vi "Result Calculation.vi"(10 "Frequency List":T1(array[cluster]), 11 "Fundamental-Response":T2(graph) caption="Fundamental-Response Mic1") -> (2 "Sensitivity Frequency (Hz)":dbl, 3 "Sensitivity (dBSPL)":dbl, 5 "Processed Freq Response":T2(graph) caption="Fundamental-Response Mic1", 7 "ProcessedFrequencyResponse":dbl[](array[numeric]))   [LabVIEW 2018]
panel:
  # "Result Calculation"
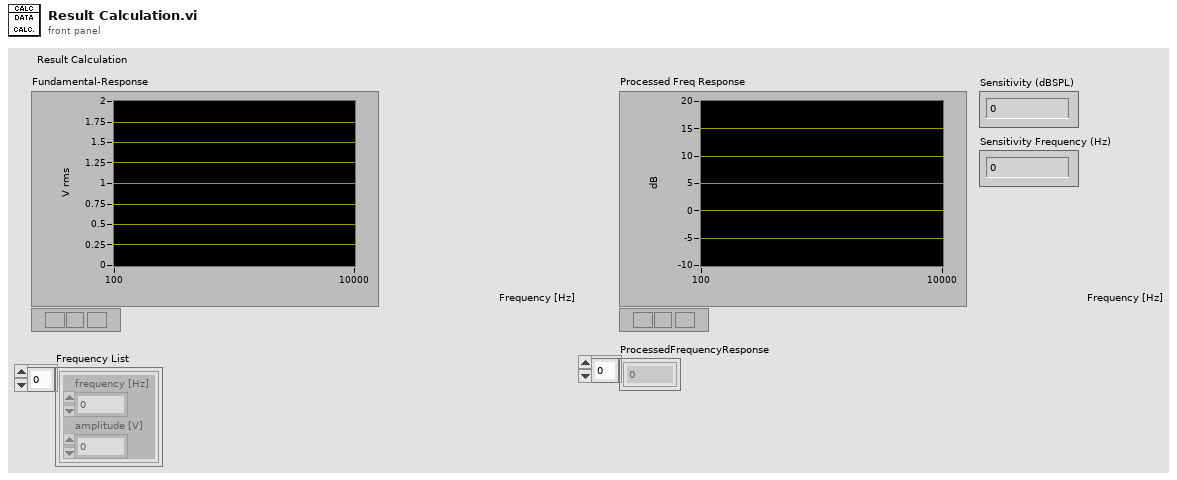
[diagram p1: front panel]
types:
  T1 = cluster{"frequency [Hz]":dbl, "amplitude [V]":dbl}[]
  T2 = cluster{"frequency [Hz]":dbl[], "amplitude":dbl[]}
  T3 = cluster{"frequency [Hz]":dbl[], "ProcessedFrequencyResponse":dbl[]}
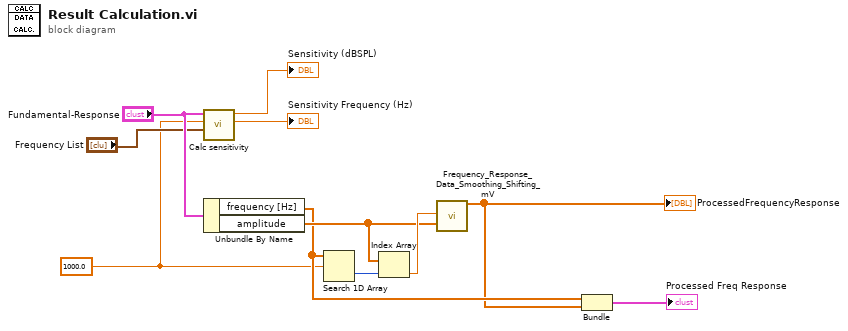
[diagram p0: block diagram]
diagram:
  w1 = 1000.0 ("element")
  n1 = call "Calc sensitivity.vi"("Frequency list Adjusted"="Frequency List", "Frequency [Hz]"=w1, "Fundamental Response"="Fundamental-Response") -> ("Sensitivity Frequency (Hz)"=→"Sensitivity Frequency (Hz)":dbl, "Sensitivity (mV/Pa)"=→"Sensitivity (dBSPL)":dbl)  [unwired: 6 in, 1 out]
  n2 = Unbundle By Name("Fundamental-Response") -> ("frequency [Hz]"=w8:dbl[], "amplitude"=w9:dbl[])
  n3 = Search 1D Array(1D array=w8, element=w1) -> (index of element=w11:i32)  [unwired: 1 in]
  n4 = Index Array(array=w9, index=w11) -> (element=w10:dbl)
  n5 = call "Frequency_Response_Data_Smoothing_Shifting_mV.vi"("Parameters.RefAmplitude"=w10, "Parameters.UUTResponseLevel.amplitude"=w9) -> ("ProcessedFrequencyResponse"=w7:dbl[])  [unwired: 17 in]
  "ProcessedFrequencyResponse" <- w7
  n6 = Bundle("frequency [Hz]"=w8, "ProcessedFrequencyResponse"=w7) -> (→"Processed Freq Response":T3)  [unwired: 1 in]
